vi "CalMic-Restore Defaults.vi"(0 "config":path) -> (8 "Params":T1)   [LabVIEW 2020]
uses:
  CalMic-Params.ctl
panel:
  in  "Error In":errorcluster
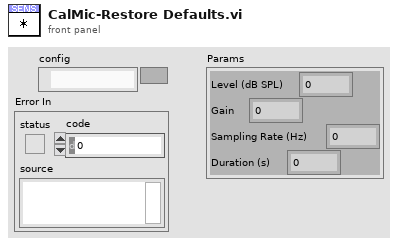
[diagram p1: front panel]
types:
  T1 = typedef "CalMic-Params.ctl" = cluster{"Level (dB SPL)":dbl, "Gain":dbl, "Sampling Rate (Hz)":dbl, "Duration (s)":dbl}
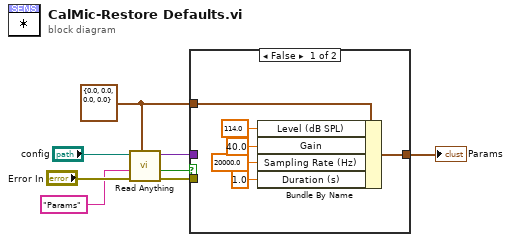
[diagram p0: block diagram]
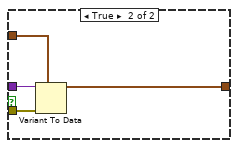
[diagram p2: hidden frame]
diagram:
  w2 = T1 {"Level (dB SPL)"=0.0, "Gain"=0.0, "Sampling Rate (Hz)"=0.0, "Duration (s)"=0.0} ("Params")
  n1 = call "Read Anything.vi"("Type of Anything"=w2, "Error In"="Error In", "Section Name (Name of \"Type of Anything\")"="Params" ("Section Name (Name of \"Type of Anything\")"), "Path (dialog)"="config") -> ("Error Out"=w5:errorcluster, "Found?"=w4:bool, "Anything"=w3:variant)  [unwired: 5 in]
  n2 = case shown="False" w4 {
    tunnel: w5 -> [_ w18]
    tunnel: w3 -> [_ w17]
    tunnel: w2 -> [w14 w16]
    tunnel: [w9 w15] -> w1
    frame False {
      n3 = Bundle By Name(cluster=w14, "Level (dB SPL)"=114.0, "Gain"=40.0, "Sampling Rate (Hz)"=20000.0, "Duration (s)"=1.0) -> (w9:T1)
    }
    frame True {
      n4 = Variant To Data(error in=w18, type=w16, Variant=w17) -> (data=w15:T1)  [unwired: 1 out]
    }
  }
  "Params" <- w1
